vi "PDF Creation.vi"() -> ()   [LabVIEW 2024]
uses:
  <vilib>/sklein/WebView2/Webview2 Control/WebView2 Control.xctl
  <vilib>/sklein/WebView2/Libs/Microsoft.Web.WebView2.Core.dll
panel:
  in  "stop":bool
  out "Timeout":bool
  in  "PDF":bool
  in  "String":string
  in  "WebView2 Control":string(xcontrol)
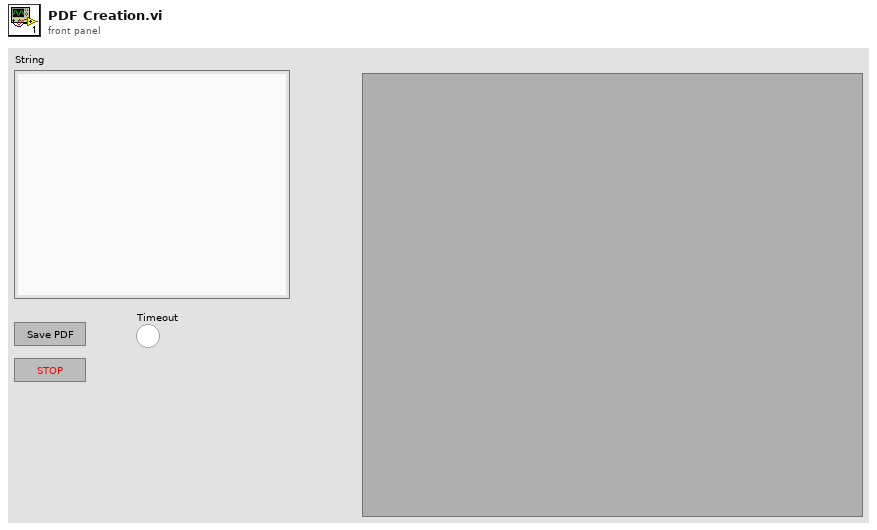
[diagram p1: front panel]
types:
  T1 = cluster{"search string":string, "replace string (\"\")":string}[]
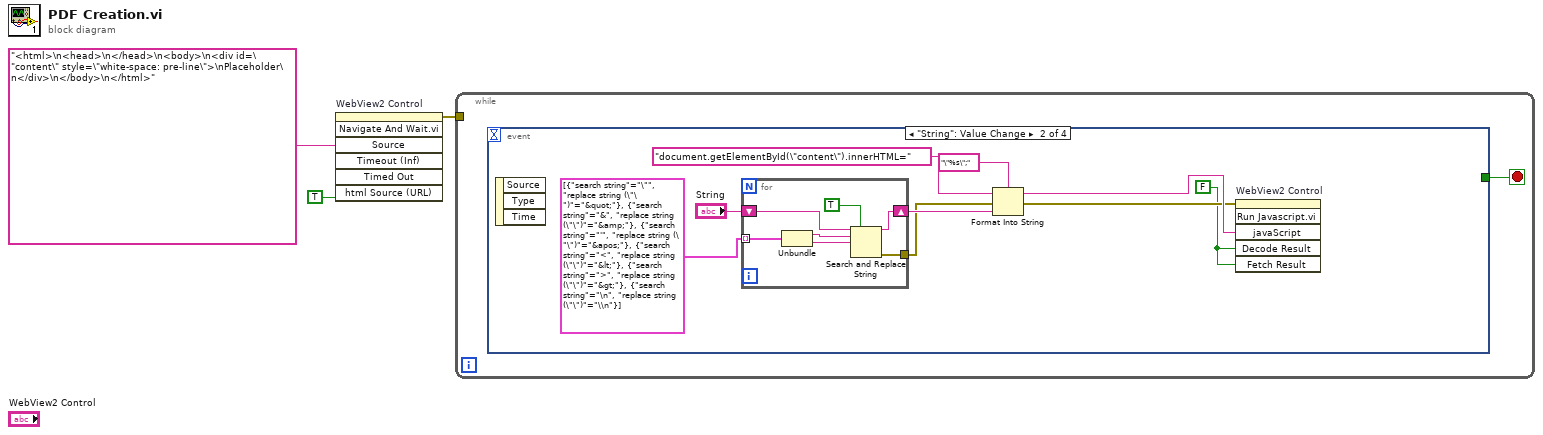
[diagram p0: block diagram]
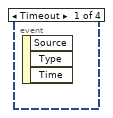
[diagram p2: hidden frame]
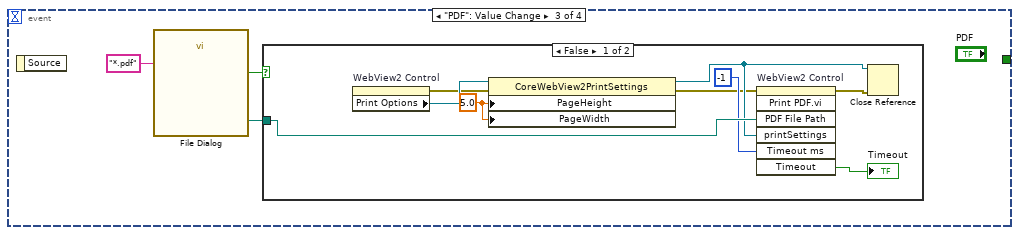
[diagram p3: hidden frame]
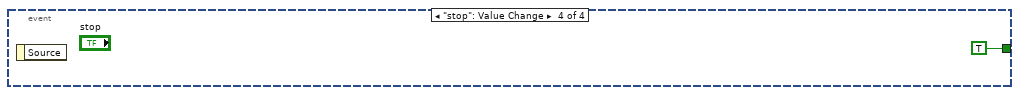
[diagram p5: hidden frame]
diagram:
  n1 = invoke on="WebView2 Control" class="WebView2 Control (strict)" method="Navigate And Wait.vi"("Source"="<html>\n<head>\n</head>\n<body>\n<div id=\"content\" style=\"white-space: pre-line\">\nPlaceholder\n</div>\n</body>\n</html>", "html Source (URL)"=TRUE) -> (error out=w1:errorcluster)  [unwired: 5 in, 6 out]
  n2 = while {
    tunnel: w1 -> [_]
    stop <- w4 stop-if-true
    n3 = event shown="[1] \"String\": Value Change" {
      selector: _ -> [_ _ _ _]
      dyn-events: _ -> [_ _ _ _]
      timeout: _ -> [_ _ _ _]
      tunnel: [_ _ _ TRUE] -> w4
      event Timeout {
        n4 = event-data() -> ()  [unwired: 1 in, 3 out]
      }
      event "String": Value Change {
        w6 = FALSE ("Decode Result")
        n5 = event-data() -> ()  [unwired: 1 in, 3 out]
        n6 = for {
          tunnel: [w17] -> w8
          shift-right: [w19] -> w9
          shift-left: "String" -> [w20]
          tunnel: T1 [{"search string"="\"", "replace string (\"\")"="&quot;"}, {"search string"="&", "replace string (\"\")"="&amp;"}, {"search string"="'", "replace string (\"\")"="&apos;"}, {"search string"="<", "replace string (\"\")"="&lt;"}, {"search string"=">", "replace string (\"\")"="&gt;"}, {"search string"="\n", "replace string (\"\")"="\\n"}] -> [w16] mode=indexing
          n7 = Unbundle(w16) -> ("search string"=w15:string, "replace string (\"\")"=w14:string)
          n8 = Search and Replace String(replace all?=TRUE ("replace all? (F)"), input string=w20, search string=w15, replace string=w14) -> (result string=w19:string, error out=w17:errorcluster)  [unwired: 4 in, 2 out]
        }
        n9 = Format Into String(format string="\"%s\";", initial string="document.getElementById(\"content\").innerHTML=" ("javaScript"), error in=w8, w9) -> (resulting string=w12:string, error out=w7:errorcluster)
        n10 = invoke on="WebView2 Control" class="WebView2 Control (strict)" method="Run Javascript.vi"(error in=w7, "javaScript"=w12, "Decode Result"=w6, "Fetch Result"=w6) -> ()  [unwired: 2 in, 6 out]
      }
      event "PDF": Value Change {
        n11 = event-data() -> ()  [unwired: 1 in, 1 out]
        n12 = call "File Dialog"("pattern (all files)"="*.pdf") -> ("selected path"=w22:path, "cancelled"=w21:bool)  [unwired: 11 in, 2 out]
        n13 = case shown="False" w21 {
          tunnel: w22 -> [w32 _]
          frame False {
            w26 = 5.0 ("PageHeight")
            n14 = property on="WebView2 Control" class="WebView2 Control (strict)"() -> (error out=w25:errorcluster, "Print Options"=w28:refnum<k24>)  [unwired: 2 in, 1 out]
            n15 = property class="CoreWebView2PrintSettings"(reference=w28, error in=w25, "PageHeight"=w26, "PageWidth"=w26) -> (reference out=w27:refnum<k24>, error out=w24:errorcluster)
            n16 = invoke on="WebView2 Control" class="WebView2 Control (strict)" method="Print PDF.vi"(error in=w24, "PDF File Path"=w32, "printSettings"=w27, "Timeout ms"=-1) -> (error out=w29:errorcluster, "Timeout"=→"Timeout":bool)  [unwired: 3 in, 5 out]
            n17 = Close Reference(reference=w27, error in (no error)=w29) -> ()  [unwired: 1 out]
          }
          frame True {
          }
        }
      }
      event "stop": Value Change {
        n18 = event-data() -> ()  [unwired: 1 in, 1 out]
      }
    }
  }
